vi "ilemt_ui.vi"() -> ()   [LabVIEW 2026]
doc: "The main user interface to the ILEMT magnetic position tracker."
uses:
  gui/display_source.ctl
  calibration/calibration.ctl
  gui/measurements.ctl
  processing/ilemt_config.ctl
  system/IO_params.ctl
  processing/stft_params.ctl
  <vilib>/Analysis/4window.llb/windowTd.ctl
  processing/filter_params.ctl
  processing/detrend_mode.ctl
  processing/modulation_info.ctl
  gui/trace_stats.ctl
  gui/frequency_display_tabs.ctl
  gui/offline_options.ctl
  gui/axis_name.ctl
  gui/levels_selector.ctl
  gui/Level selector 1.ctl
  gui/Level selector 4.ctl
  gui/Level selector 3.ctl
  gui/Level selector 2.ctl
  gui/spectrum_parameters.ctl
  gui/output_options.ctl
  gui/coupling_selector.ctl
  main/ilemt_status.ctl
  gui/display_options.ctl
  main/ilemt_globals.vi
  <vilib>/Analysis/NI_AALPro.lvlib
panel:
  in  "Log demod":bool=TRUE
  in  "Log raw":bool=TRUE
  out "Low drive":bool
  in  "Amplitude/phase":bool
  in  "Display card":enum16{"Current", "Sensor"}(ring)=enum."Sensor" caption="Card"
  in  "Reset RMS":bool
  in  "AC/DC":bool
  in  "Clipping":bool
  in  "Source axis":T1
  out "Measurements":T2 {"RMS" format="%#_3p"; "Relative" format="%.4f"; "Ref distance" format="%.3f"; "DC" format="%.3f"}
  in  "Output options":enum32{"Levels", "Offline", "Options"}(tab)
  out "Levels 2":dbl[][](array[numeric]) caption="Levels 1" format="%.3f"
  in  "Levels selector 2":T3={"Signal source"=enum."Carrier levels", "Mode"=enum."Phase", "re."=enum."Ref level", "High/low"=enum."High", "Sense"=TRUE}
  in  "Levels selector 1":T3={"Signal source"=enum."Trace display", "Mode"=enum."dB", "re."=enum."Full scale", "High/low"=enum."High", "Sense"=FALSE}
  out "Levels 1":dbl[][](array[numeric]) format="%.3f"
  out "Replaying":bool
  in  "Offline options":T8 {"Range" min=0 step=1}
  out "Current":i32
  in  "Offline size":i32=150
  in  "Source/sensor selection":T9={"Source"=enum."Vector", "Sensor"=enum."Vector", "Sense"=TRUE, "Distance"=TRUE, "LF corner"=0.2, "RMS Tc"=20.0}
  out "Logging":bool
  in  "Start Logging":bool
  in  "Stop Logging":bool
  in  "Log File":path
  out "Backlog":bool
  in  "Sensor axis":T1
  out "NaN":bool
  in  "Stop":bool=TRUE
  out "Offline (hidden)":bool
  in  "Frequency display":T11
  out "Spectrum":waveform(dbl)[](graph)
  in  "Full spectrum":bool
  in  "Low spectrum":bool
  in  "High spectrum":bool
  in  "Restart Averaging":bool
  in  "Spectrum parameters":T12={"Window"=enum."7 Term B-Harris", "FFT blocking"=enum."2", "Averaging"=2.0, "Order"=8} {"Order" min=1 max=100; "Averaging" min=0.0 max=1000.0 step=1.0}
  in  "Demod spectrum":bool
  out "STFT Spectrogram":dbl[][](graph)
  in  "Map selector":T13(ring)=enum."rainbow"
  out "Autocorrelation":dbl[](graph)
  out "AC max XY":dbl[](array[numeric]) caption="Max correlation"
  out "Time dom stats":T14 {"dB" format="%.1f"; "RMS" format="%#_3p"; "DC" format="%#_3p"; "|max|" format="%#_3p"}
  out "Config (hidden)":T15={"IO params"={"Conversion"={"Rate"=0.0, "Num cards"=0, "Out channels"=4}, "Carriers"={"Phase shift"=180.0, "Levels"=[[0.8, 0.8, 0.8], [0.03, 0.03, 0.03]], "Delay samples"=73.15}, "TCP"={"Host"="192.168.1.15", "Port"=6666, "Buffering"=6, "Timeout"=6}, "Input channel sign"=[1, 1, 1]}, "High rate STFT"={"Win param"=0.0, "Window type"=0, "Win order"=0, "DFT size"=0, "Channels"=[], "Oversample"=0}, "Low rate STFT"={"Win param"=0.0, "Window type"=0, "Win order"=0, "DFT size"=0, "Channels"=[], "Oversample"=0}, "Filtering "=[]} {"Filtering"."Distortion"."Limit" format="%#_3p"; "Filtering"."Distortion"."LF cut" format="%#_3p"; "Filtering"."Kalman"."Measure noise" format="%#_3p"; "Filtering"."Kalman"."Process noise" format="%#_3p"; "Filtering"."Hum"."Limit" format="%#_3p"; "Filtering"."Hum"."Frequency" format="%#_4p"; "Low rate STFT"."Oversample" min=1 step=1; "Low rate STFT"."Channels" min=0 step=1; "Low rate STFT"."DFT size" min=1 step=1; "Low rate STFT"."Window type" items=["Rectangle"=0, "Hanning"=1, "Hamming"=2, "Blackman-Harris"=3, "Exact Blackman"=4, "Blackman"=5, "Flat Top"=6, "4 Term B-Harris "=7, "7 Term B-Harris"=8, "Low Sidelobe"=9, "Blackman Nuttall"=11, "Triangle"=30, "Bartlett-Hanning"=31, "Bohman"=32, "Parzen"=33, "Welch"=34, "Kaiser"=60, "Dolph-Chebyshev"=61, "Gaussian"=62]; "High rate STFT"."Oversample" min=1 step=1; "High rate STFT"."Channels" min=0 step=1; "High rate STFT"."DFT size" min=1 step=1; "High rate STFT"."Window type" items=["Rectangle"=0, "Hanning"=1, "Hamming"=2, "Blackman-Harris"=3, "Exact Blackman"=4, "Blackman"=5, "Flat Top"=6, "4 Term B-Harris "=7, "7 Term B-Harris"=8, "Low Sidelobe"=9, "Blackman Nuttall"=11, "Triangle"=30, "Bartlett-Hanning"=31, "Bohman"=32, "Parzen"=33, "Welch"=34, "Kaiser"=60, "Dolph-Chebyshev"=61, "Gaussian"=62]; "IO params"."Input channel sign" min=-1 max=1 step=1; "IO params"."Carriers"."Levels" min=0.0 step=0.1; "IO params"."Conversion"."Rate" format="%#_8g"}
  in  "Set ref":bool
  in  "Settings":T21(tab)
  out "6DOF cal OK":bool caption="OK"
  in  "6DOF calibration":path=path "C:/Users/robma/Documents/Work/ilemt_cal_data/cal_9_24_premo_rotated_dipole/foo.cal"
  in  "Reference calibration":bool
  in  "Calibrate":bool
  in  "Cal data":dbl[][](array[numeric])=[[0.04, 0.1443141016057697, 0.0003271339007519708], [0.03, 0.3386348577606244, 0.0007671086833412981], [0.05, 0.07397569851632148, 0.000167769359644626], [0.07, 0.027209296148070442, 6.176768913465489e-05]] format="%#_4f"
  out "RMS error":dbl format="%_3p"
  out "Residuals":dbl[](array[numeric]) format="%_3p"
  out "Cal status":bool
  out "Calibration":T22={"Ks"=[9.043189074449675e-06, 6.83137056161437e-08], "r bias"=-8.410156592895371e-05} {"r bias" format="%_3p"; "Ks" format="%#_3p"}
  in  "Range (mm)":dbl=0.07
  in  "Clear cal":bool
  in  "Solve":bool
  in  "Freq response cal":bool
  in  "Coupling signs":i32[](array[numeric])=[-1, -1, 1] min=-1 max=1 step=1
  in  "Filtering":T19[](array[typedef])=[{"Hum"={"Frequency"=60.0, "Tc"=0.3, "Limit"=0.001, "FFT filter"=FALSE, "Detrend mode"=enum."Robust linear", "Enable"=FALSE}, "Kalman"={"Process noise"=3e-05, "Measure noise"=0.0003}, "Distortion"={"LF cut"=0.0, "Tc"=1.0, "Limit"=0.001, "FFT filter"=FALSE, "Detrend mode"=enum."Linear", "Enable"=TRUE}}, {"Hum"={"Frequency"=60.0, "Tc"=0.3, "Limit"=0.001, "FFT filter"=FALSE, "Detrend mode"=enum."Robust linear", "Enable"=FALSE}, "Kalman"={"Process noise"=0.0001, "Measure noise"=6e-05}, "Distortion"={"LF cut"=0.0, "Tc"=1.0, "Limit"=0.0003, "FFT filter"=FALSE, "Detrend mode"=enum."Robust linear", "Enable"=TRUE}}] {"Distortion"."Limit" format="%#_3p"; "Distortion"."LF cut" format="%#_3p"; "Kalman"."Measure noise" format="%#_3p"; "Kalman"."Process noise" format="%#_3p"; "Hum"."Limit" format="%#_3p"; "Hum"."Frequency" format="%#_4p"}
  out "Source waveforms":waveform(dbl)[](graph)
  in  "IO params":T16={"Conversion"={"Rate"=48828.125, "Num cards"=2, "Out channels"=4}, "Carriers"={"Phase shift"=180.0, "Levels"=[[0.4, 0.4, 0.4], [0.1, 0.1, 0.1]], "Delay samples"=73.15}, "TCP"={"Host"="192.168.1.15", "Port"=6666, "Buffering"=10, "Timeout"=2000}, "Input channel sign"=[1, 1, 1]} {"Input channel sign" min=-1 max=1 step=1; "Carriers"."Levels" min=0.0 step=0.1; "Conversion"."Rate" format="%#_8g"}
  out "I RMS":dbl[](array[numeric]) format="%.3g"
  out "Comp fault":bool
  in  "Input card":i32=1 min=0 max=3 step=1
  in  "Always display":bool
  out "Read backlog":i32
  out "Restart IO":bool
  out "Modulation info":T23={"Fs full"=0.0, "Fs high"=0.0, "Fs low"=0.0, "Read size"=5000, "FFT size low"=5000, "df low"=5000.0, "High carriers"=[], "Low carriers"=[], "Hi channels at low"=[7]} {"Hi channels at low" min=0 step=1; "Low carriers" format="%#_6p"; "High carriers" format="%#_6p"}
  in  "Low rate STFT":T17={"Win param"=0.0, "Window type"=3, "Win order"=2, "DFT size"=8192, "Channels"=[46, 56, 62], "Oversample"=2} {"Oversample" min=1 step=1; "Channels" min=0 step=1; "DFT size" min=1 step=1; "Window type" items=["Rectangle"=0, "Hanning"=1, "Hamming"=2, "Blackman-Harris"=3, "Exact Blackman"=4, "Blackman"=5, "Flat Top"=6, "4 Term B-Harris "=7, "7 Term B-Harris"=8, "Low Sidelobe"=9, "Blackman Nuttall"=11, "Triangle"=30, "Bartlett-Hanning"=31, "Bohman"=32, "Parzen"=33, "Welch"=34, "Kaiser"=60, "Dolph-Chebyshev"=61, "Gaussian"=62]}
  in  "High rate STFT":T17={"Win param"=0.0, "Window type"=1, "Win order"=2, "DFT size"=32, "Channels"=[5, 7, 9], "Oversample"=1} {"Oversample" min=1 step=1; "Channels" min=0 step=1; "DFT size" min=1 step=1; "Window type" items=["Rectangle"=0, "Hanning"=1, "Hamming"=2, "Blackman-Harris"=3, "Exact Blackman"=4, "Blackman"=5, "Flat Top"=6, "4 Term B-Harris "=7, "7 Term B-Harris"=8, "Low Sidelobe"=9, "Blackman Nuttall"=11, "Triangle"=30, "Bartlett-Hanning"=31, "Bohman"=32, "Parzen"=33, "Welch"=34, "Kaiser"=60, "Dolph-Chebyshev"=61, "Gaussian"=62]}
  out "Noise delta":dbl[][](array[numeric]) format="%.1f"
  out "Noise floor":dbl[][](array[numeric]) format="%.1f"
  in  "Noise ref":bool
  out "Chart":waveform(dbl)[](graph)
  out "Mean level (hidden)":dbl[](array[numeric])
  in  "stop":bool
  in  "Display signal":T24 caption="Signal"
  out "Time domain":waveform(dbl)[](graph)
  # "Input"
  # "Output"
  # "Z    Y    X"
  # "Source"
  # "X                 Y                 Z"
  # "Sensor"
  # "Start"
  # "End"
  # "1DOF calibration"
  # "Range"
  # "Levels"
  # "High"
  # "Low"
  # "X"
  # "Y"
  # "Z"
  # "High"
  # "Low"
  # "X"
  # "Y"
  # "Z"
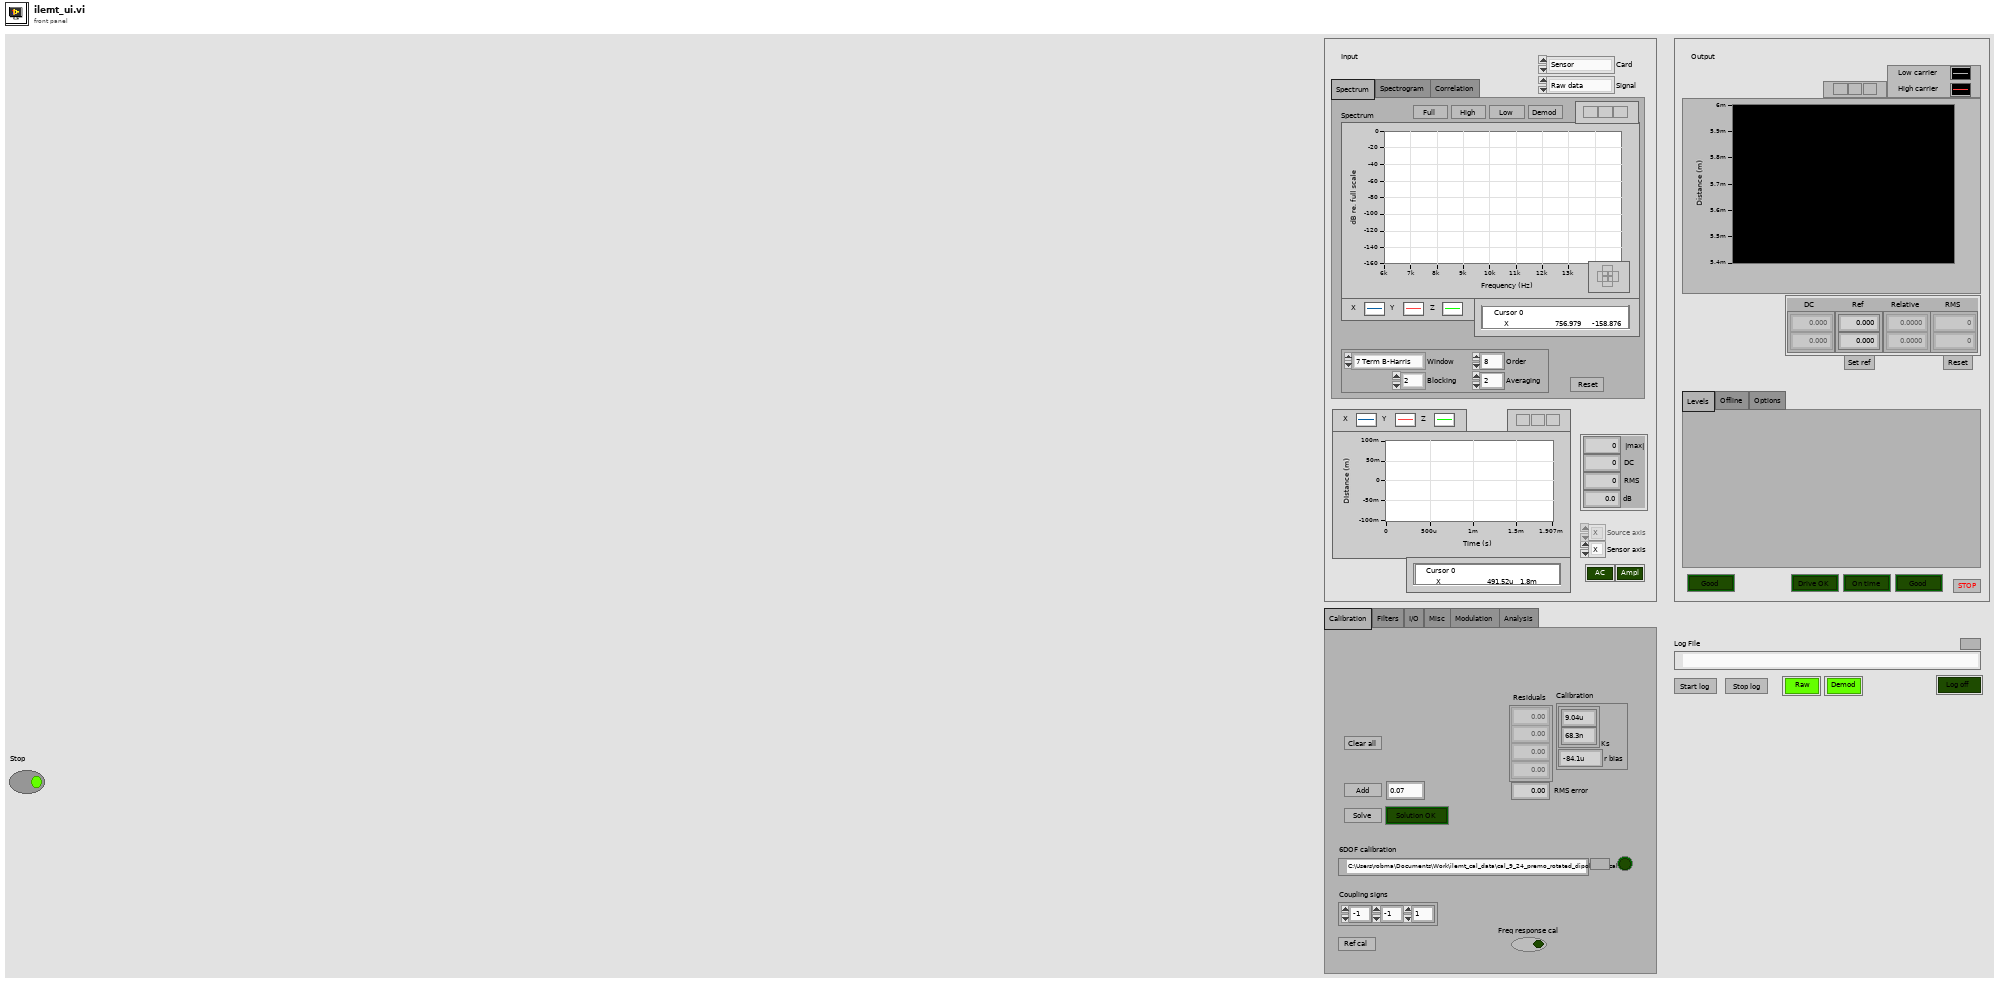
[diagram p1: front panel]
types:
  T1 = typedef "axis_name.ctl" = enum16{"X", "Y", "Z"}
  T2 = typedef "measurements.ctl" = cluster{"DC":dbl[], "Ref distance":dbl[], "Relative":dbl[], "RMS":dbl[]}
  T3 = typedef "levels_selector.ctl" = cluster{"Signal source":T4, "Mode":T5, "re.":T6, "High/low":T7, "Sense":bool}
  T4 = typedef "Level selector 1.ctl" = enum16{"Trace display", "Carrier levels", "Ref levels"}
  T5 = typedef "Level selector 4.ctl" = enum16{"Level", "dB", "Phase", "Mismatch"}
  T6 = typedef "Level selector 3.ctl" = enum16{"Full scale", "Carrier", "Ref level", "Noise"}
  T7 = typedef "Level selector 2.ctl" = enum16{"High", "Low"}
  T8 = typedef "offline_options.ctl" = cluster{"Offline":bool, "Trigger":bool, "Range":i32[], "Run mode":enum32{"Run", "Step"}}
  T9 = typedef "output_options.ctl" = cluster{"Source":T10, "Sensor":T10, "Sense":bool, "Distance":bool, "LF corner":dbl, "RMS Tc":dbl}
  T10 = typedef "coupling_selector.ctl" = enum16{"X", "Y", "Z", "Vector"}
  T11 = typedef "frequency_display_tabs.ctl" = enum32{"Spectrum", "Spectrogram", "Correlation"}
  T12 = typedef "spectrum_parameters.ctl" = cluster{"Window":enum16{"None ", "Hanning", "Hamming", "Blackman-Harris", "Exact Blackman", "Blackman", "Flat Top", "4 Term B-Harris ", "7 Term B-Harris", "Low Sidelobe"}, "FFT blocking":enum16{"1", "2", "4", "8"}, "Averaging":dbl, "Order":u32}
  T13 = enum16{"fire", "rainbow", "grey", "inverse grey", "ice", "original"}
  T14 = typedef "trace_stats.ctl" = cluster{"|max|":dbl, "DC":dbl, "RMS":dbl, "dB":dbl}
  T15 = typedef "ilemt_config.ctl" = cluster{"IO params":T16, "High rate STFT":T17, "Low rate STFT":T17, "Filtering ":T19[]}
  T16 = typedef "IO_params.ctl" = cluster{"Conversion":cluster{"Rate":dbl, "Num cards":u32, "Out channels":u32}, "Carriers":cluster{"Phase shift":dbl, "Levels":dbl[][], "Delay samples":dbl}, "TCP":cluster{"Host":string, "Port":i32, "Buffering":u32, "Timeout":u32}, "Input channel sign":i32[]}
  T17 = typedef "stft_params.ctl" = cluster{"Win param":dbl, "Window type":T18, "Win order":i32, "DFT size":i32, "Channels":i32[], "Oversample":i32}
  T18 = typedef "NI_AALPro.lvlib/windowTd.ctl" = u32
  T19 = typedef "filter_params.ctl" = cluster{"Hum":cluster{"Frequency":dbl, "Tc":dbl, "Limit":dbl, "FFT filter":bool, "Detrend mode":T20, "Enable":bool}, "Kalman":cluster{"Process noise":dbl, "Measure noise":dbl}, "Distortion":cluster{"LF cut":dbl, "Tc":dbl, "Limit":dbl, "FFT filter":bool, "Detrend mode":T20, "Enable":bool}}
  T20 = typedef "detrend_mode.ctl" = enum16{"Zero mean", "Linear", "Robust linear"}
  T21 = enum32{"Calibration", "Filters", "I/O", "Misc", "Modulation", "Analysis"}
  T22 = typedef "calibration.ctl" = cluster{"Ks":dbl[], "r bias":dbl}
  T23 = typedef "modulation_info.ctl" = cluster{"Fs full":dbl, "Fs high":dbl, "Fs low":dbl, "Read size":i32, "FFT size low":i32, "df low":dbl, "High carriers":dbl[], "Low carriers":dbl[], "Hi channels at low":i32[]}
  T24 = typedef "display_source.ctl" = enum16{"Raw data", "Carrier predict", "Residue", "STFT low", "STFT high", "KF input", "KF output", "KF noise", "Distortion", "Hum", "Distance high", "Chart high", "Chart low"}
  T25 = typedef "ilemt_status.ctl" = cluster{"NaN":bool, "Backlog":bool, "Clipping":bool}
  T26 = typedef "trace_info.ctl" = cluster{"Channels":T27[][], "Chart data":waveform(dbl)[][], "Distance high":dbl[], "Status":T25}
  T27 = typedef "trace_channel.ctl" = cluster{"Raw data":dbl[], "Carrier prediction":dbl[], "Residue":dbl[], "STFT low":cdb[], "STFT high":cdb[][], "KF input":cdb[][], "KF outupt":cdb[][], "KF noise":dbl[][], "Distortion":cdb[][], "Hum":cdb[][]}
  T28 = typedef "high_carrier_amplitudes.ctl" = cdb[][][][]
  T29 = typedef "carrier_amplitudes.ctl" = cdb[][][][]
  T30 = typedef "display_options.ctl" = cluster{"Display card":i32, "Signal":T24, "Source axis":T1, "Sensor axis":T1, "Spectrum parameters":T12, "AC/DC":bool, "Amplitude/Phase":bool, "Levels selectors":T3[], "Map selector":enum16{"fire", "rainbow", "grey", "inverse grey", "ice", "original"}, "Restart Averaging":bool, "Noise ref":bool}
  T31 = cluster{"Autocorrelation":dbl[], "AC max XY":dbl[]}
  T32 = cluster{"Noise floor":dbl[][], "Noise delta":dbl[][]}
  T33 = enum8{"Enabled", "Disabled", "Disabled and Grayed Out"}
  T34 = typedef "6dof_calibration.ctl" = cluster{"d_source_pos":dbl[][], "d_source_moment":dbl[][], "d_sensor_pos":dbl[][], "d_sensor_moment":dbl[][], "linear_correction":dbl[][]}
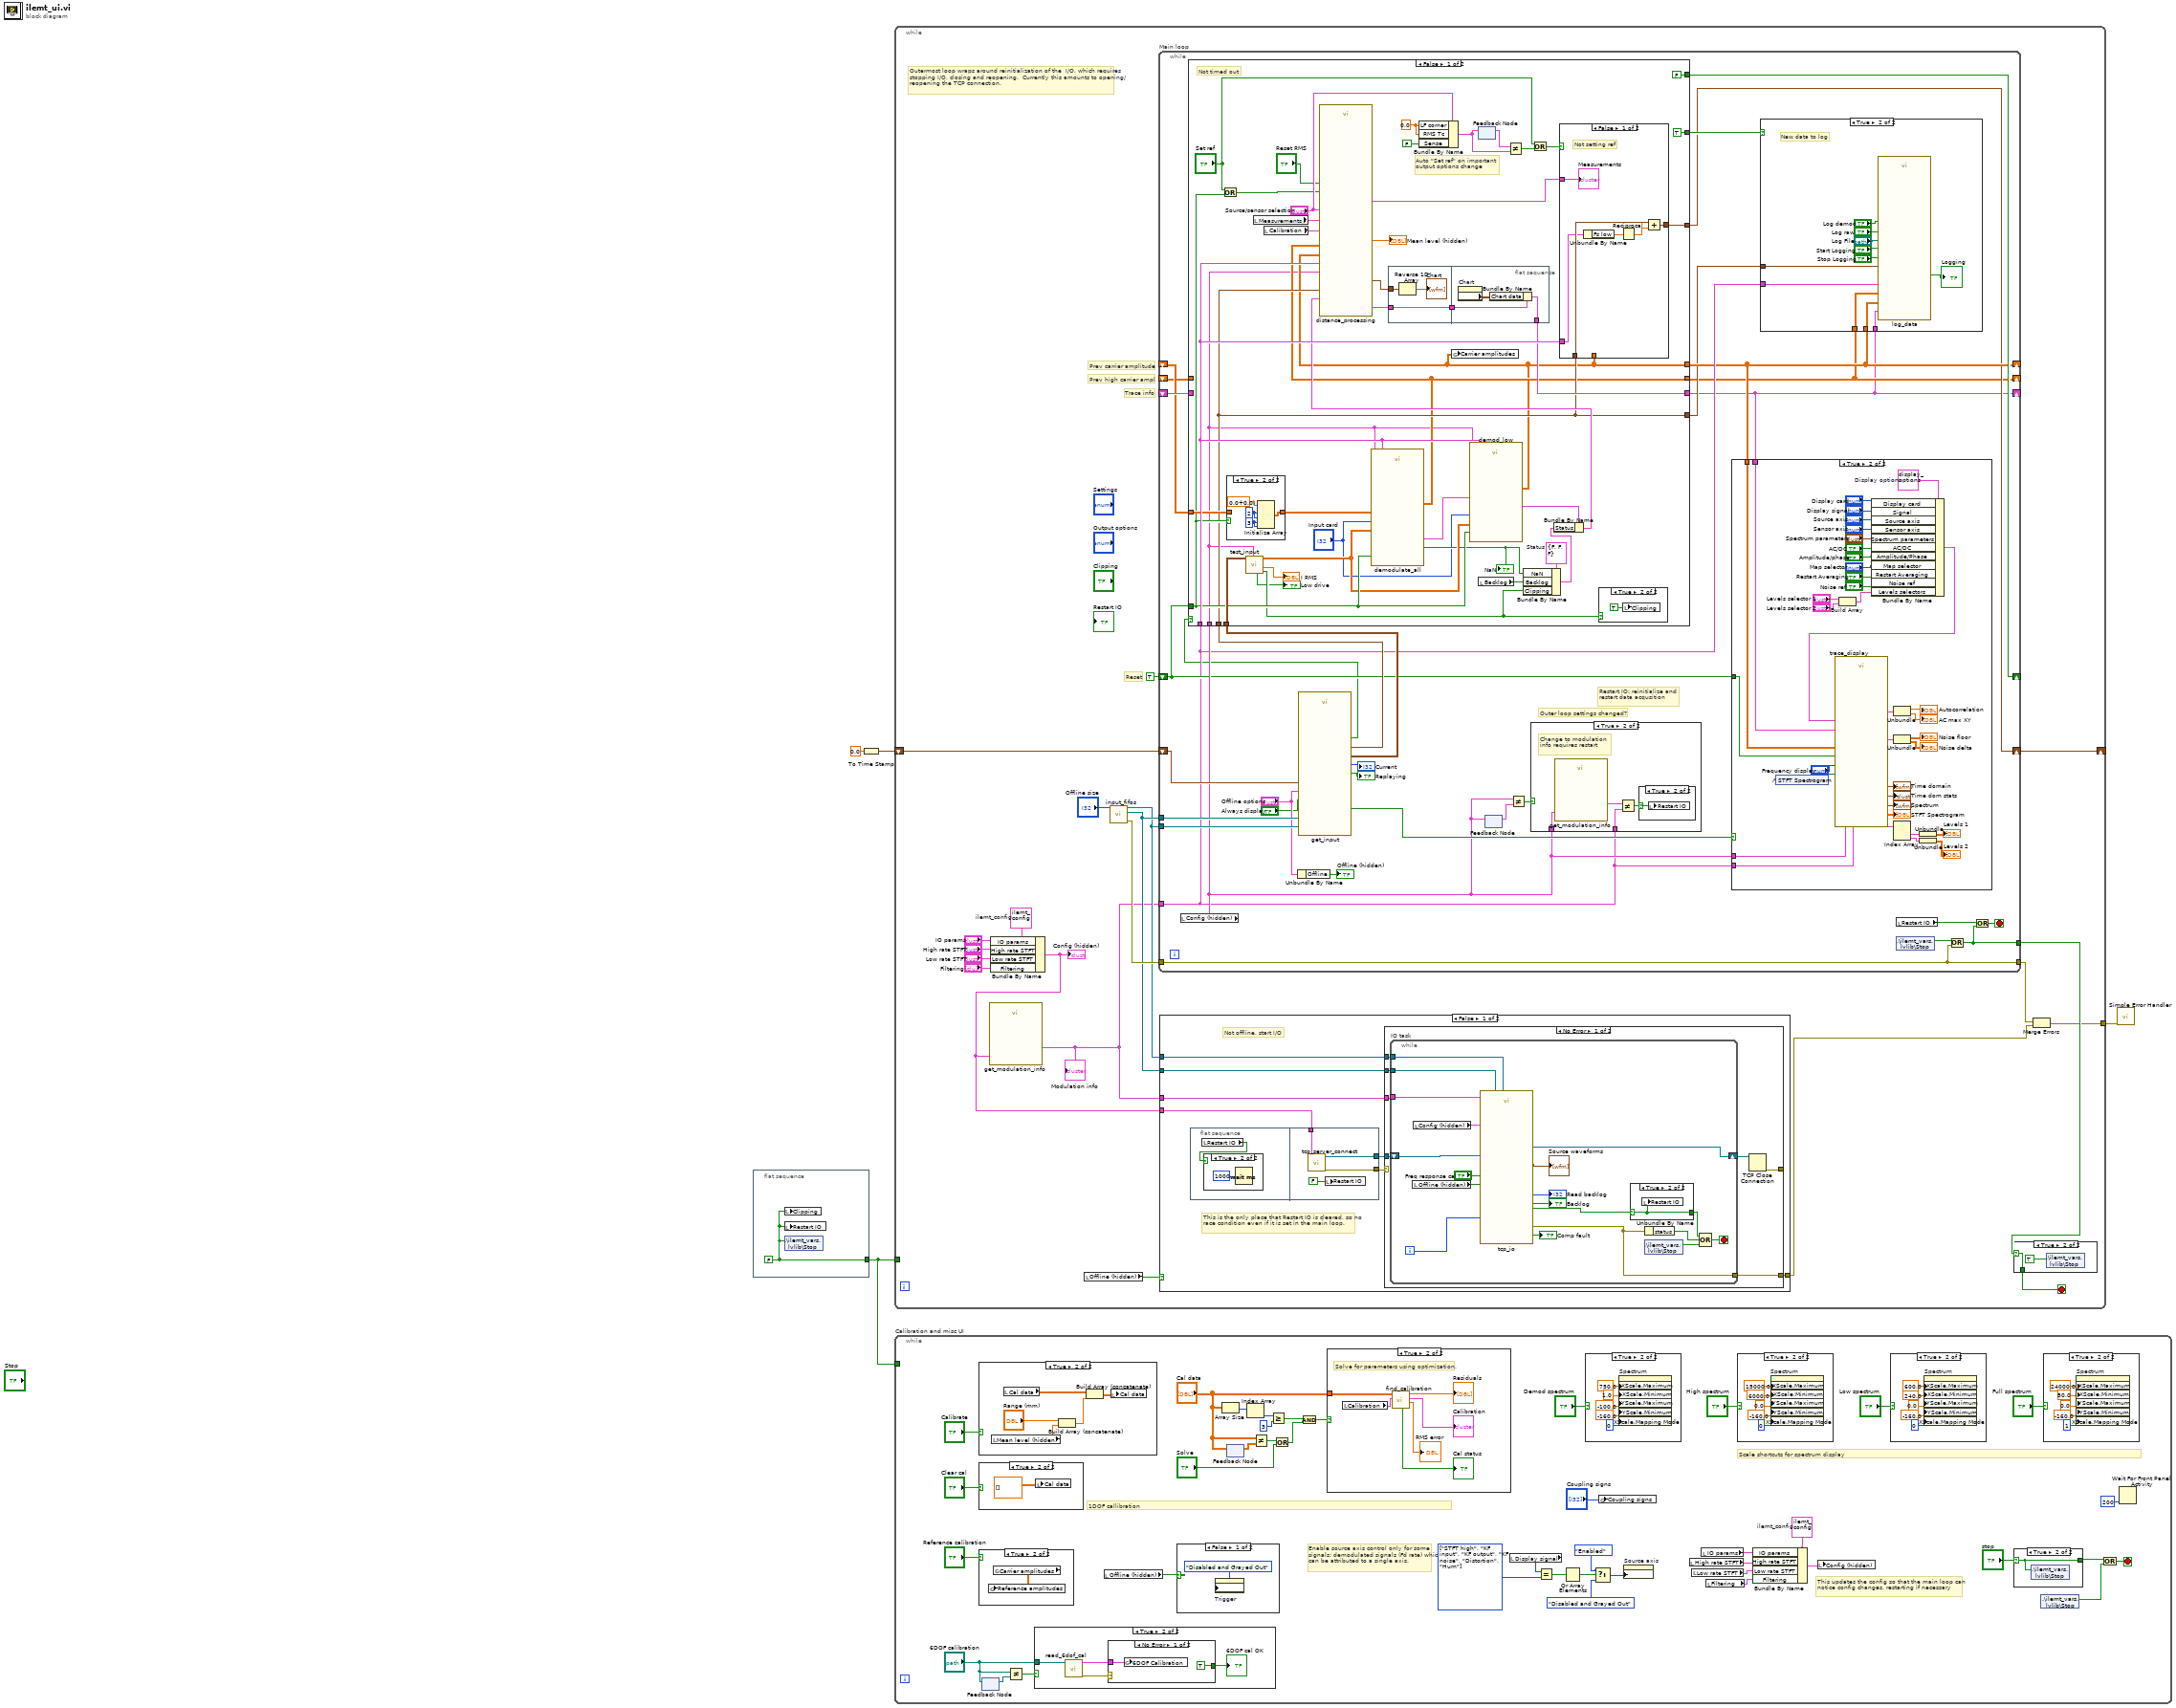
[diagram p0: block diagram]
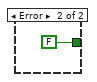
[diagram p3: hidden frame]
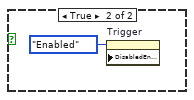
[diagram p6: hidden frame]
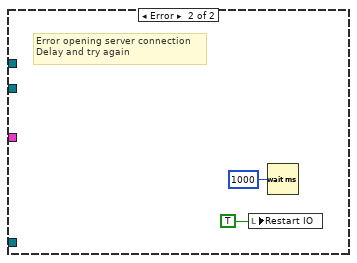
[diagram p15: hidden frame]
diagram:
  n1 = flat-sequence {
    tunnel: [w5] -> w4
    frame #0 {
      w5 = FALSE ("stop")
      n2 = local write "Clipping"(w5) -> ()
      n3 = local write "Restart IO"(w5) -> ()
      n4 = shared-variable ".\\ilemt_vars.lvlib\\Stop"(w5) -> ()  [unwired: 1 in, 1 out]
    }
  }
  n5 = To Time Stamp(1:0.0 ("Fs low")) -> (0:w2:timestamp)
  n6 = while {
    tunnel: w4 -> [_]
    shift-right: [w22] -> _
    shift-left: w2 -> [w23]
    tunnel: [w7] -> w1
    stop <- w10 stop-if-true
    w13 = T15 {"IO params"={"Conversion"={"Rate"=0.0, "Num cards"=0, "Out channels"=4}, "Carriers"={"Phase shift"=180.0, "Levels"=[[0.8, 0.8, 0.8], [0.03, 0.03, 0.03]], "Delay samples"=73.15}, "TCP"={"Host"="192.168.1.15", "Port"=6666, "Buffering"=6, "Timeout"=6}, "Input channel sign"=[1, 1, 1]}, "High rate STFT"={"Win param"=0.0, "Window type"=0, "Win order"=0, "DFT size"=0, "Channels"=[], "Oversample"=0}, "Low rate STFT"={"Win param"=0.0, "Window type"=0, "Win order"=0, "DFT size"=0, "Channels"=[], "Oversample"=0}, "Filtering "=[]}  # ilemt_config
    # "Prev high carrier ampl"
    # "Prev carrier amplitude"
    # "Trace info"
    # "Outermost loop wraps around reinitialization of the  I/O, which requires stopping I/O, closing and reopening.  Currently this amounts to opening/reopening the TCP connection."
    # "Reset"
    n7 = Bundle By Name(cluster=w13, "IO params"="IO params", "High rate STFT"="High rate STFT", "Low rate STFT"="Low rate STFT", "Filtering"="Filtering") -> (w11:T15)
    "Config (hidden)" <- w11
    n8 = call "get_modulation_info.vi"("Config"=w11) -> ("Modulation info"=w6:T23)  [unwired: 10 in]
    "Modulation info" <- w6
    n9 = local read "Offline (hidden)"() -> (w14:bool)
    n10 = call "input_fifos.vi"("Offline size"="Offline size") -> ("error out"=w21:errorcluster, "queue out 2"=w20:refnum<queue>, "Queue out"=w15:refnum<queue>)  [unwired: 8 in]
    n11 = while "Main loop" {
      tunnel: w21 -> [w81]
      tunnel: [w103] -> w24
      tunnel: w6 -> [w82]
      shift-right: [w96] -> _
      shift-left: TRUE -> [w87]
      tunnel: [w81] -> w9
      shift-right: [w77] -> w22
      shift-left: w23 -> [w98]
      tunnel: w20 -> [w101]
      shift-right: [w78] -> _
      shift-left: _ -> [w84]
      tunnel: w15 -> [w99]
      shift-right: [w72] -> _
      shift-left: _ -> [w85]
      shift-right: [w75] -> _
      shift-left: _ -> [w74]
      stop <- w102 stop-if-true
      # "Restart IO: reinitialize and restart data acqusition"
      # "Outer loop settings changed?"
      # "Read Sound Data"
      n12 = local read "Config (hidden)"() -> (w92:T15)
      n13 = Unbundle By Name("Offline options") -> ("Offline"=→"Offline (hidden)":bool)
      n14 = call "get_input.vi"("Offline queue"=w99, "Read queue"=w101, "Offline options"="Offline options", "Time Stamp in"=w98, "Always display"="Always display") -> ("timed out?"=w79:bool, "Input data"=w100:waveform(dbl)[][], "Current"=→"Current":i32, "Time Stamp out"=w88:timestamp, "Display update"=w95:bool, "Replaying"=→"Replaying":bool)  [unwired: 5 in]
      n15 = case shown="False" w79 {
        tunnel: [FALSE w230] -> w96
        tunnel: w87 -> [w179 w230]
        tunnel: w92 -> [w157 _]
        tunnel: [w193 w226] -> w77
        tunnel: w82 -> [w190 _]
        tunnel: w100 -> [w192 _]
        tunnel: w84 -> [w183 w229]
        tunnel: [w160 w229] -> w78
        tunnel: [w188 w228] -> w72
        tunnel: w85 -> [_ w228]
        tunnel: w88 -> [w163 w226]
        tunnel: [TRUE FALSE] -> w83
        tunnel: [w163 w226] -> w76
        tunnel: [w162 w225] -> w75
        tunnel: w74 -> [_ w225]
        frame False {
          w172 = T25 {"NaN"=FALSE, "Backlog"=FALSE, "Clipping"=FALSE}  # Status
          w176 = 0.0 ("LF corner")
          # "Auto \"Set ref\" on important output options change"
          # "Not timed out"
          n16 = Or(x="Set ref", y=w179) -> (x .or. y?=w174:bool)
          n17 = case shown="True" w179 {
            tunnel: [w200 w202] -> w184
            tunnel: w183 -> [w200 _]
            frame False {
            }
            frame True {
              w201 = 3 ("dimension size")
              w204 = 2 ("dimension size")
              n18 = Initialize Array(cdb 0.0+0.0i, w204, w204, w201, w201) -> (w202:cdb[][][][])
            }
          }
          n19 = call "test_input.vi"("Config"=w157, "data in"=w192) -> ("Clipping"=w165:bool, "I RMS"=→"I RMS":dbl[], "Raw data"=w167:dbl[][][], "Drive low"=→"Low drive":bool)  [unwired: 6 in]
          n20 = local read "Measurements"() -> (w195:T2)
          n21 = local read "Calibration"() -> (w197:T22)
          n22 = call "demodulate_all.vi"("Config"=w157, "Prev carrier amplitudes"=w184, "Input card"="Input card", "Modulation info"=w190, "Reset"=w179, "Raw data"=w167) -> ("Trace info out"=w191:T26, "High carrier amplitudes"=w162:T28, "NaN"=w166:bool)  [unwired: 3 in]
          "NaN" <- w166
          n23 = flat-sequence {
            tunnel: w189 -> [w207]
            tunnel: [w207] -> w187
            tunnel: w186 -> [w205]
            tunnel: [w208] -> w188
            tunnel: w187 -> [w210]
            frame #0 {
              n24 = Reverse 1D Array(array=w205) -> (reversed array=→"Chart":waveform(dbl)[])
            }
            frame #1 {
              n25 = property on="Chart" class="WFChart (strict)"() -> ("History Data"=w209:waveform(dbl)[][])  [unwired: 2 in, 2 out]
              n26 = Bundle By Name(cluster=w210, "Chart data"=w209) -> (w208:T26)
            }
          }
          n27 = Bundle By Name(cluster="Source/sensor selection", "LF corner"=w176, "RMS Tc"=w176, "Sense"=FALSE) -> (w177:T9)
          n28 = call "demod_low.vi"("Reset"=w179, "Config"=w157, "Modulation info"=w190, "Input card"="Input card", "Trace info in"=w191, "Raw data"=w167) -> ("Carrier amplitudes"=w160:T29, "Trace info out"=w170:T26)  [unwired: 8 in]
          n29 = global write "ilemt_globals.vi" "Carrier amplitudes"(w160) -> ()
          n30 = feedback-in #1(w177) -> ()
          n31 = feedback #1() -> (w181:T9)  [unwired: 1 in]
          n32 = local read "Backlog"() -> (w173:bool)
          n33 = Not Equal?(x=w181, y=w177) -> (x != y?=w158:bool)
          n34 = Bundle By Name(cluster=w172, "NaN"=w166, "Backlog"=w173, "Clipping"=w165) -> (w171:T25)
          n35 = Or(x="Set ref", y=w158) -> (x .or. y?=w180:bool)
          n36 = Bundle By Name(cluster=w170, "Status"=w171) -> (w169:T26)
          n37 = call "distance_processing.vi"("Trace info in"=w169, "Time Stamp"=w163, "Config"=w157, "Carrier amplitudes"=w160, "Output options"="Source/sensor selection", "Modulation info"=w190, "Calibration"=w197, "Reset"=w174, "Reset RMS"="Reset RMS", "Measurements In"=w195, "High carrier amplitudes"=w162) -> ("Measurements out"=w185:T2, "Mean level"=→"Mean level (hidden)":dbl[], "Chart display"=w186:waveform(dbl)[], "Trace info out"=w189:T26)  [unwired: 13 in]
          n38 = case shown="False" w180 {
            tunnel: w163 -> [w214 _]
            tunnel: [w213 w222] -> w193
            tunnel: w190 -> [w212 _]
            tunnel: w160 -> [_ w217]
            tunnel: w185 -> [w211 w219]
            frame False {
              # "Not setting ref"
              n39 = Unbundle By Name(w212) -> ("Fs low"=w216:dbl)
              n40 = Reciprocal(x=w216) -> (1/x=w215:dbl)
              n41 = Add(x=w214, y=w215) -> (x+y=w213:timestamp)
              "Measurements" <- w211
            }
            frame True {
              # "Set ref"
              # "Zero time"
              # "Clear chart"
              n42 = Unbundle By Name(w219) -> ("DC"=w221:dbl[])
              n43 = local write "Clipping"(FALSE ("Clipping")) -> ()
              n44 = global write "ilemt_globals.vi" "GUI reference"(w217) -> ()
              n45 = Bundle By Name(cluster=w219, "Ref distance"=w221) -> (w220:T2)
              n46 = local write "Measurements"(w220) -> ()
              n47 = property on="Chart" class="WFChart (strict)"("History Data"=waveform(dbl)[][] [] ("Chart")) -> ()  [unwired: 2 in, 2 out]
              n48 = To Time Stamp(1:0.0 ("Fs low")) -> (0:w222:timestamp)
            }
          }
          n49 = case shown="True" w165 {
            frame False {
            }
            frame True {
              n50 = local write "Clipping"(TRUE ("Clipping")) -> ()
            }
          }
        }
        frame True {
          # "Queue read timed out.  Just try again, unless the portents say it's time to exit."
        }
      }
      n51 = feedback-in #2(w92) -> ()
      n52 = feedback #2() -> (w94:T15)  [unwired: 1 in]
      n53 = Not Equal?(x=w92, y=w94) -> (x != y?=w93:bool)
      n54 = case shown="True" w93 {
        tunnel: w92 -> [_ w118]
        tunnel: w82 -> [_ w116]
        frame False {
        }
        frame True {
          # "Change to modulation info requires restart"
          n55 = call "get_modulation_info.vi"("Config"=w118) -> ("Modulation info"=w117:T23)  [unwired: 10 in]
          n56 = Not Equal?(x=w117, y=w116) -> (x != y?=w115:bool)
          n57 = case shown="True" w115 {
            selector: w115 -> [_ w119]
            frame False {
            }
            frame True {
              n58 = local write "Restart IO"(w119) -> ()
            }
          }
        }
      }
      n59 = case shown="True" w95 {
        tunnel: w92 -> [_ w155]
        tunnel: w82 -> [_ w154]
        tunnel: w87 -> [_ w134]
        tunnel: w78 -> [_ w151]
        tunnel: w72 -> [_ w150]
        frame False {
        }
        frame True {
          w135 = T30 {"Display card"=0, "Signal"=enum."Raw data", "Source axis"=enum."X", "Sensor axis"=enum."X", "Spectrum parameters"={"Window"=enum."7 Term B-Harris", "FFT blocking"=enum."2", "Averaging"=2.0, "Order"=8}, "AC/DC"=FALSE, "Amplitude/Phase"=FALSE, "Levels selectors"=[{"Signal source"=enum."Trace display", "Mode"=enum."dB", "re."=enum."Full scale", "High/low"=enum."High", "Sense"=FALSE}, {"Signal source"=enum."Carrier levels", "Mode"=enum."Phase", "re."=enum."Ref level", "High/low"=enum."High", "Sense"=TRUE}], "Map selector"=enum."rainbow", "Restart Averaging"=FALSE, "Noise ref"=FALSE}  # Display options
          n60 = control-ref of="STFT Spectrogram"() -> (w153:refnum<vi>)
          n61 = Build Array("Levels selector 1", "Levels selector 2") -> (w146:T3[])
          n62 = Bundle By Name(cluster=w135, "Display card"="Display card", "Signal"="Display signal", "Source axis"="Source axis", "Sensor axis"="Sensor axis", "Spectrum parameters"="Spectrum parameters", "AC/DC"="AC/DC", "Amplitude/Phase"="Amplitude/phase", "Map selector"="Map selector", "Restart Averaging"="Restart Averaging", "Noise ref"="Noise ref", "Levels selectors"=w146) -> (w133:T30)
          n63 = call "trace_display.vi"("Carrier amplitudes"=w151, "Frequency display"="Frequency display", "Spectrogram reference"=w153, "Config"=w155, "Reset"=w134, "Modulation info"=w154, "Display options"=w133, "Trace info"=w150) -> ("Autocorrelation"=w127:T31, "Levels arrays"=w128:cluster{"Levels":dbl[][]}[], "STFT Spectrogram"=→"STFT Spectrogram":dbl[][], "Time domain"=→"Time domain":waveform(dbl)[], "Time statistics"=→"Time dom stats":T14, "Spectrum"=→"Spectrum":waveform(dbl)[], "Noise"=w124:T32)  [unwired: 13 in]
          n64 = Unbundle(w127) -> ("Autocorrelation"=→"Autocorrelation":dbl[], "AC max XY"=→"AC max XY":dbl[])
          n65 = Unbundle(w124) -> ("Noise floor"=→"Noise floor":dbl[][], "Noise delta"=→"Noise delta":dbl[][])
          n66 = Index Array(array=w128) -> (element #1=w130:cluster{"Levels":dbl[][]}, element #2=w129:cluster{"Levels":dbl[][]})  [unwired: 2 in]
          n67 = Unbundle(w130) -> ("Levels"=→"Levels 1":dbl[][])
          n68 = Unbundle(w129) -> ("Levels"=→"Levels 2":dbl[][])
        }
      }
      n69 = case shown="True" w83 {
        tunnel: w76 -> [_ w114]
        tunnel: w82 -> [_ w109]
        tunnel: w78 -> [_ w108]
        tunnel: w75 -> [_ w107]
        tunnel: w72 -> [_ w106]
        frame False {
        }
        frame True {
          # "New data to log"
          n70 = call "log_data.vi"("Log File"="Log File", "Carrier amplitudes"=w108, "Log raw"="Log raw", "Log demod"="Log demod", "Start Logging"="Start Logging", "High carrier amplitudes"=w107, "Stop Logging"="Stop Logging", "Timestamp"=w114, "Trace info"=w106, "Modulation info"=w109) -> ("Logging"=→"Logging":bool)  [unwired: 5 in]
        }
      }
      n71 = local read "Restart IO"() -> (w73:bool)
      n72 = shared-variable ".\\ilemt_vars.lvlib\\Stop"() -> (w80:bool)  [unwired: 1 in, 1 out]
      n73 = Or(x=w80, y=w81) -> (x .or. y?=w103:bool)
      n74 = Or(x=w73, y=w103) -> (x .or. y?=w102:bool)
    }
    n75 = case shown="False" w14 {
      tunnel: w6 -> [w30 _]
      tunnel: w20 -> [w32 _]
      tunnel: w15 -> [w31 _]
      tunnel: [w29 _] -> w8
      tunnel: w11 -> [w28 _]
      frame False {
        # "This is the only place that Restart IO is cleared, so no race condition even if it is set in the main loop."
        # "Not offline, start I/O"
        n76 = flat-sequence {
          tunnel: w28 -> [w67]
          tunnel: [w66] -> w27
          tunnel: [w65] -> w26
          frame #0 {
            n77 = local read "Restart IO"() -> (w63:bool)
            n78 = case shown="True" w63 {
              frame False {
              }
              frame True {
                n79 = Wait (ms)(milliseconds to wait=u32 1000) -> ()  [unwired: 1 out]
              }
            }
          }
          frame #1 {
            n80 = call "tcp_server_connect.vi"("Config"=w67) -> ("error out"=w65:errorcluster, "connection ID"=w66:refnum<k5>)  [unwired: 9 in]
            n81 = local write "Restart IO"(FALSE ("Restart IO")) -> ()
          }
        }
        n82 = case shown="No Error" w26 {
          tunnel: w32 -> [w39 _]
          tunnel: w31 -> [w38 _]
          tunnel: w30 -> [w37 _]
          tunnel: [w36 _] -> w29
          tunnel: w27 -> [w35 _]
          tunnel: [w33 _] -> _
          frame No Error {
            n83 = while "IO task" {
              tunnel: w39 -> [w57]
              tunnel: [w45] -> w36
              tunnel: w38 -> [w56]
              tunnel: w37 -> [w53]
              shift-right: [w41] -> w34
              shift-left: w35 -> [w44]
              i -> [w52]
              stop <- w58 stop-if-true
              n84 = local read "Offline (hidden)"() -> (w50:bool)
              n85 = local read "Config (hidden)"() -> (w51:T15)
              n86 = call "tcp_io.vi"("Offline queue"=w56, "Modulation info"=w53, "Config"=w51, "Read queue"=w57, "Freq response"="Freq response cal", "Connection in"=w44, "Write sequence"=w52, "Offline"=w50) -> ("Read backlog"=→"Read backlog":i32, "Backlog"=→"Backlog":bool, "Connection out"=w41:refnum<k5>, "Source waveforms"=→"Source waveforms":waveform(dbl)[], "Restart IO"=w43:bool, "Comp fault"=→"Comp fault":bool, "error out"=w45:errorcluster)  [unwired: 1 in]
              n87 = case shown="True" w43 {
                selector: w43 -> [w59 w60]
                tunnel: [w59 w60] -> w42
                frame False {
                }
                frame True {
                  n88 = local write "Restart IO"(w60) -> ()
                }
              }
              n89 = Unbundle By Name(w45) -> ("status"=w55:bool)
              n90 = shared-variable ".\\ilemt_vars.lvlib\\Stop"() -> (w54:bool)  [unwired: 1 in, 1 out]
              n91 = Compound Arithmetic op=OR(w42, w55, w54) -> (w58:bool)
            }
            n92 = TCP Close Connection(connection ID=w34) -> (error out=w33:errorcluster)  [unwired: 2 in, 1 out]
          }
          frame Error {
            # "Error opening server connection\nDelay and try again"
            n93 = local write "Restart IO"(TRUE ("Restart IO")) -> ()
            n94 = Wait (ms)(milliseconds to wait=u32 1000) -> ()  [unwired: 1 out]
          }
        }
      }
      frame True {
        # "If offline at start, don't try to start I/O.  This allows us to work in offline mode w/o hardware."
      }
    }
    n95 = case shown="True" w24 {
      selector: w24 -> [w69 w71]
      tunnel: [w69 w71] -> w10
      frame False {
      }
      frame True {
        n96 = shared-variable ".\\ilemt_vars.lvlib\\Stop"(TRUE ("stop")) -> ()  [unwired: 1 in, 1 out]
      }
    }
    n97 = Merge Errors(w9, w8) -> (w7:errorcluster)
  }
  n98 = while "Calibration and misc UI" {
    tunnel: w4 -> [_]
    stop <- w239 stop-if-true
    w238 = T24[] [enum."STFT high", enum."KF input", enum."KF output", enum."KF noise", enum."Distortion", enum."Hum"] items=["Raw data", "Carrier predict", "Residue", "STFT low", "STFT high", "KF input", "KF output", "KF noise", "Distortion", "Hum", "Distance high", "Chart high", "Chart low"]
    w248 = T15 {"IO params"={"Conversion"={"Rate"=0.0, "Num cards"=0, "Out channels"=4}, "Carriers"={"Phase shift"=180.0, "Levels"=[[0.8, 0.8, 0.8], [0.03, 0.03, 0.03]], "Delay samples"=73.15}, "TCP"={"Host"="192.168.1.15", "Port"=6666, "Buffering"=6, "Timeout"=6}, "Input channel sign"=[1, 1, 1]}, "High rate STFT"={"Win param"=0.0, "Window type"=0, "Win order"=0, "DFT size"=0, "Channels"=[], "Oversample"=0}, "Low rate STFT"={"Win param"=0.0, "Window type"=0, "Win order"=0, "DFT size"=0, "Channels"=[], "Oversample"=0}, "Filtering "=[]}  # ilemt_config
    # "1DOF callibration"
    # "Scale shortcuts for spectrum display"
    # "This updates the config so that the main loop can notice config changes, restarting if necessary"
    # "Enable source axis control only for some signals: demodulated signals (Fd rate) which can be attributed to a single axis."
    n99 = case shown="True" "Calibrate" {
      frame False {
      }
      frame True {
        n100 = local read "Mean level (hidden)"() -> (w310:dbl[])
        n101 = local read "Cal data"() -> (w312:dbl[][])
        n102 = Build Array (concatenate)("Range (mm)", w310) -> (w313:dbl[])
        n103 = Build Array (concatenate)(w312, w313) -> (w311:dbl[][])
        n104 = local write "Cal data"(w311) -> ()
      }
    }
    n105 = case shown="True" "Clear cal" {
      frame False {
      }
      frame True {
        n106 = local write "Cal data"(dbl[][] [] ("Cal data")) -> ()
      }
    }
    n107 = case shown="True" "Reference calibration" {
      frame False {
      }
      frame True {
        n108 = global read "ilemt_globals.vi" "Carrier amplitudes"() -> (w283:T29)
        n109 = global write "ilemt_globals.vi" "Reference amplitudes"(w283) -> ()
      }
    }
    n110 = feedback #3() -> (w233:path)  [unwired: 1 in]
    n111 = feedback-in #3("6DOF calibration") -> ()
    n112 = Not Equal?(x="6DOF calibration", y=w233) -> (x != y?=w232:bool)
    n113 = case shown="True" w232 {
      tunnel: "6DOF calibration" -> [_ w274]
      frame False {
      }
      frame True {
        n114 = call "read_6dof_cal.vi"("Path"=w274) -> ("error out"=w273:errorcluster, "6DOF Calibration"=w272:T34)  [unwired: 9 in]
        n115 = case shown="No Error" w273 {
          tunnel: w272 -> [w276 _]
          tunnel: [TRUE ("6DOF cal OK") FALSE ("6DOF cal OK")] -> w271
          frame No Error {
            n116 = global write "ilemt_globals.vi" "6DOF Calibration"(w276) -> ()
          }
          frame Error {
          }
        }
        "6DOF cal OK" <- w271
      }
    }
    n117 = local read "Offline (hidden)"() -> (w237:bool)
    n118 = case shown="False" w237 {
      frame False {
        n119 = property on="Trigger" class="Bool"("DisabledEnum"=T33."Disabled and Grayed Out" ("Disabled")) -> ()  [unwired: 2 in, 2 out]
      }
      frame True {
        n120 = property on="Trigger" class="Bool"("DisabledEnum"=T33."Enabled" ("Disabled")) -> ()  [unwired: 2 in, 2 out]
      }
    }
    n121 = Array Size(array="Cal data") -> (size(s)=w247:i32[])
    n122 = feedback-in #4("Cal data") -> ()
    n123 = feedback #4() -> (w269:dbl[][])  [unwired: 1 in]
    n124 = Index Array(array=w247) -> (element=w245:i32)  [unwired: 1 in]
    n125 = Not Equal?(x="Cal data", y=w269) -> (x != y?=w267:bool)
    n126 = Greater Or Equal?(x=w245, y=3) -> (x >= y?=w243:bool)
    n127 = Or(x=w267, y="Solve") -> (x .or. y?=w265:bool)
    n128 = And(x=w243, y=w265) -> (x .and. y?=w264:bool)
    n129 = case shown="True" w264 {
      tunnel: "Cal data" -> [_ w304]
      frame False {
      }
      frame True {
        # "Solve for parameters using optimization."
        n130 = local read "Calibration"() -> (w309:T22)
        n131 = call "find_calibration.vi"("Calibration in"=w309, "Cal data"=w304) -> ("f(minimum)"=→"RMS error":dbl, "Calibration out"=→"Calibration":T22, "Residuals"=→"Residuals":dbl[], "status"=→"Cal status":bool)  [unwired: 6 in]
      }
    }
    n132 = local read "Display signal"() -> (w254:T24)
    n133 = Equal?(x=w254, y=w238) -> (x = y?=w253:bool[])
    n134 = Or Array Elements(Boolean array=w253) -> (logical OR=w250:bool)
    n135 = case shown="True" "Demod spectrum" {
      frame False {
      }
      frame True {
        n136 = property on="Spectrum" class="WFGraph (strict)"("XScale.Maximum"=750.0 ("X Scale.Range:Maximum"), "XScale.Minimum"=1.0 ("X Scale.Range:Minimum"), "YScale.Maximum"=-100.0 ("Y Scale.Range:Maximum"), "YScale.Minimum"=-160.0 ("Y Scale.Range:Minimum"), "XScale.Mapping Mode"=u8 0 ("X Scale.Mapping Mode")) -> ()  [unwired: 2 in, 2 out]
      }
    }
    n137 = Select(t=T33."Enabled" ("Disabled"), s=w250, f=T33."Disabled and Grayed Out" ("Disabled")) -> (s? t:f=w249:T33)
    n138 = global write "ilemt_globals.vi" "Coupling signs"("Coupling signs") -> ()
    n139 = property on="Source axis" class="Enum (strict)"("DisabledEnum"=w249) -> ()  [unwired: 2 in, 2 out]
    n140 = local read "High rate STFT"() -> (w258:T17)
    n141 = local read "Low rate STFT"() -> (w257:T17)
    n142 = local read "IO params"() -> (w259:T16)
    n143 = local read "Filtering"() -> (w256:T19[])
    n144 = case shown="True" "High spectrum" {
      frame False {
      }
      frame True {
        n145 = property on="Spectrum" class="WFGraph (strict)"("XScale.Maximum"=15000.0 ("X Scale.Range:Maximum"), "XScale.Minimum"=6000.0 ("X Scale.Range:Minimum"), "YScale.Maximum"=0.0 ("Y Scale.Range:Maximum"), "YScale.Minimum"=-160.0 ("Y Scale.Range:Minimum"), "XScale.Mapping Mode"=u8 0 ("X Scale.Mapping Mode")) -> ()  [unwired: 2 in, 2 out]
      }
    }
    n146 = Bundle By Name(cluster=w248, "IO params"=w259, "High rate STFT"=w258, "Low rate STFT"=w257, "Filtering"=w256) -> (w260:T15)
    n147 = local write "Config (hidden)"(w260) -> ()
    n148 = case shown="True" "Low spectrum" {
      frame False {
      }
      frame True {
        n149 = property on="Spectrum" class="WFGraph (strict)"("XScale.Maximum"=600.0 ("X Scale.Range:Maximum"), "XScale.Minimum"=240.0 ("X Scale.Range:Minimum"), "YScale.Maximum"=0.0 ("Y Scale.Range:Maximum"), "YScale.Minimum"=-160.0 ("Y Scale.Range:Minimum"), "XScale.Mapping Mode"=u8 0 ("X Scale.Mapping Mode")) -> ()  [unwired: 2 in, 2 out]
      }
    }
    n150 = case shown="True" "stop" {
      selector: "stop" -> [w286 w287]
      tunnel: [w286 w287] -> w241
      frame False {
      }
      frame True {
        n151 = shared-variable ".\\ilemt_vars.lvlib\\Stop"(w287) -> ()  [unwired: 1 in, 1 out]
      }
    }
    n152 = shared-variable ".\\ilemt_vars.lvlib\\Stop"() -> (w240:bool)  [unwired: 1 in, 1 out]
    n153 = case shown="True" "Full spectrum" {
      frame False {
      }
      frame True {
        n154 = property on="Spectrum" class="WFGraph (strict)"("XScale.Maximum"=24000.0 ("X Scale.Range:Maximum"), "XScale.Minimum"=50.0 ("X Scale.Range:Minimum"), "YScale.Maximum"=0.0 ("Y Scale.Range:Maximum"), "YScale.Minimum"=-160.0 ("Y Scale.Range:Minimum"), "XScale.Mapping Mode"=u8 1 ("X Scale.Mapping Mode")) -> ()  [unwired: 2 in, 2 out]
      }
    }
    n155 = Or(x=w241, y=w240) -> (x .or. y?=w239:bool)
    n156 = Wait For Front Panel Activity(1:200 ("timeout ms (-1 never timeout)")) -> ()  [unwired: 2 in, 1 out]
  }
  n157 = call <vilib>:"Simple Error Handler.vi"("error in (no error)"=w1) -> ()  [unwired: 4 in, 5 out]
